vi "Usuarios-VI.vi"() -> (1 "Retroceder LED":bool, 2 "Estacionarse LED":bool)   [LabVIEW 2024]
uses:
  <vilib>/DAQmx/read.llb/DAQmx Read (Counter U32 1Chan 1Samp).vi
  <vilib>/DAQmx/miscellaneous.llb/DAQmx Fill In Error Info.vi
panel:
  in  "Retroceder":bool
  in  "Estacionarse":bool
  in  "Usuario invalido":T1={"Nombre de usuario"="Usuario NO Valido", "Nombre"="", "Fotografía"=FALSE}
  in  "Usuario 3":T1={"Nombre de usuario"="Yucateco_Belicon_27", "Nombre"="David Alejandro Zarazua Martinez", "Fotografía"=FALSE}
  in  "Usuario 1":T1={"Nombre de usuario"="Test_1", "Nombre"="Roberto Gomez Cruz", "Fotografía"=FALSE}
  in  "Usuario 2":T1={"Nombre de usuario"="El_Inge", "Nombre"="Ivan Nieto Guerrero", "Fotografía"=FALSE}
  out "Mensaje de entrada":string
  out "Credencial":u32
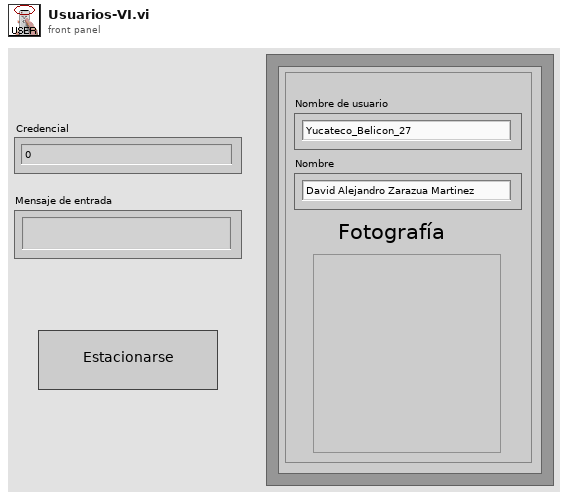
[diagram p1: front panel]
types:
  T1 = cluster{"Nombre de usuario":string, "Nombre":string, "Fotografía":bool}
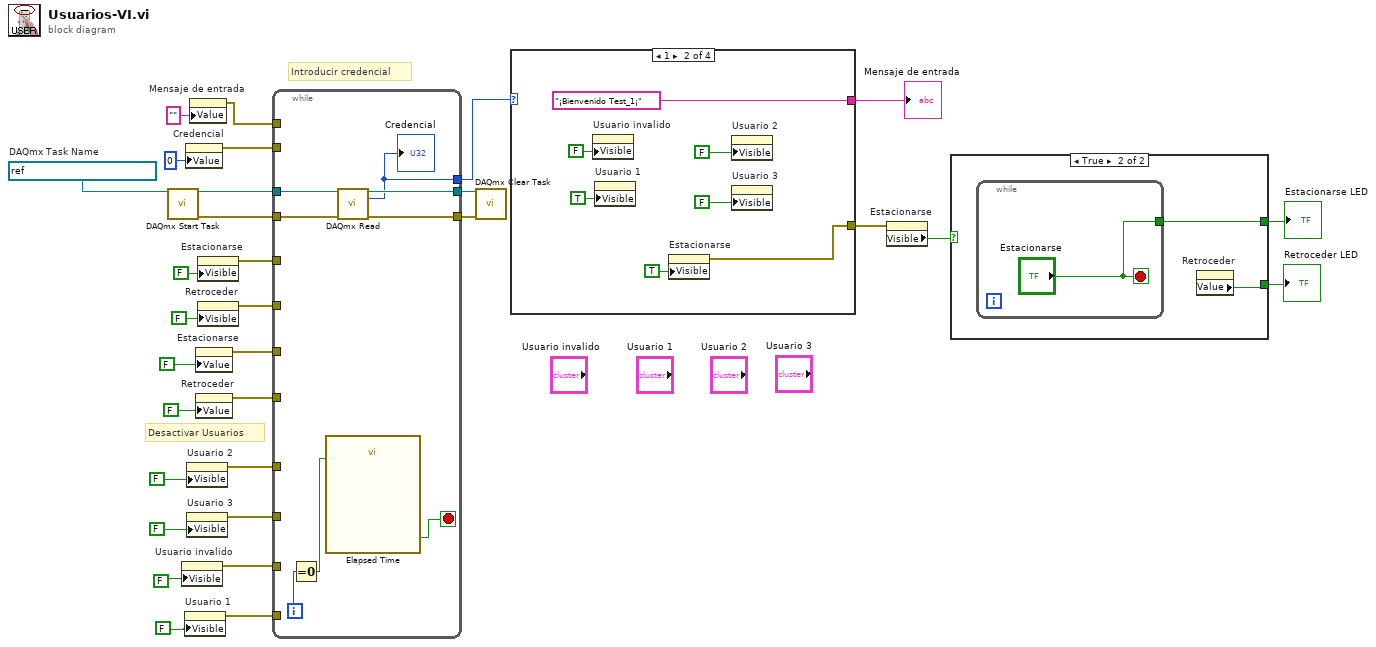
[diagram p0: block diagram]
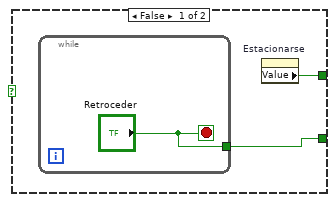
[diagram p2: hidden frame]
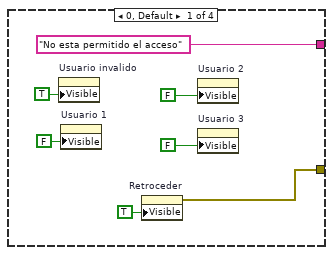
[diagram p3: hidden frame]
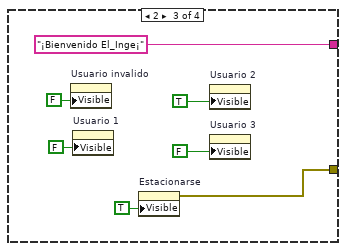
[diagram p4: hidden frame]
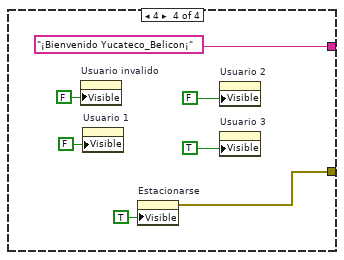
[diagram p5: hidden frame]
diagram:
  w31 = refnum<k21> "Contador de Pulso PF1"  # DAQmx Task Name
  # "Introducir credencial"
  # "Desactivar Usuarios"
  n1 = call <vilib>:"DAQmx Start Task.vi"("task/channels in"=w31) -> ("task out"=w30:refnum<k21>, "error out"=w29:errorcluster)  [unwired: 13 in]
  n2 = property on="Usuario invalido" class="Clust (strict)"("Visible"=FALSE) -> (error out=w18:errorcluster)  [unwired: 2 in, 1 out]
  n3 = property on="Usuario 1" class="Clust (strict)"("Visible"=FALSE) -> (error out=w17:errorcluster)  [unwired: 2 in, 1 out]
  n4 = property on="Credencial" class="DigNum (strict)"("Value"=u32 0 ("Credencial")) -> (error out=w14:errorcluster)  [unwired: 2 in, 1 out]
  n5 = property on="Usuario 2" class="Clust (strict)"("Visible"=FALSE) -> (error out=w23:errorcluster)  [unwired: 2 in, 1 out]
  n6 = property on="Usuario 3" class="Clust (strict)"("Visible"=FALSE) -> (error out=w24:errorcluster)  [unwired: 2 in, 1 out]
  n7 = property on="Mensaje de entrada" class="Str"("Value"="" ("Mensaje de entrada")) -> (error out=w13:errorcluster)  [unwired: 2 in, 1 out]
  n8 = property on="Estacionarse" class="Bool (strict)"("Value"=FALSE ("Estacionarse")) -> (error out=w6:errorcluster)  [unwired: 2 in, 1 out]
  n9 = property on="Retroceder" class="Bool (strict)"("Value"=FALSE ("Retroceder")) -> (error out=w5:errorcluster)  [unwired: 2 in, 1 out]
  n10 = property on="Estacionarse" class="Bool (strict)"("Visible"=FALSE) -> (error out=w8:errorcluster)  [unwired: 2 in, 1 out]
  n11 = property on="Retroceder" class="Bool (strict)"("Visible"=FALSE) -> (error out=w7:errorcluster)  [unwired: 2 in, 1 out]
  n12 = while {
    tunnel: w30 -> [w36]
    tunnel: w29 -> [w39]
    tunnel: [w37] -> w21
    tunnel: [w38] -> w20
    tunnel: [w35] -> w19
    tunnel: w24 -> [_]
    tunnel: w23 -> [_]
    tunnel: w18 -> [_]
    tunnel: w17 -> [_]
    tunnel: w14 -> [_]
    tunnel: w13 -> [_]
    tunnel: w8 -> [_]
    tunnel: w7 -> [_]
    tunnel: w6 -> [_]
    tunnel: w5 -> [_]
    i -> [w33]
    stop <- w34 stop-if-true
    n13 = Equal To 0?(x=w33) -> (x = 0?=w32:bool)
    n14 = call "Elapsed Time"("Reset"=w32) -> ("Time has Elapsed"=w34:bool)  [unwired: 11 in, 7 out]
    n15 = call-poly <vilib>:"DAQmx Read.vi"("task/channels in"=w36, "error in"=w39) -> ("task out"=w37:refnum<k21>, "data"=w35:u32, "error out"=w38:errorcluster)  [unwired: 11 in]
    "Credencial" <- w35
  }
  n16 = call <vilib>:"DAQmx Clear Task.vi"("task in"=w21, "error in"=w20) -> ()  [unwired: 13 in, 1 out]
  n17 = case shown="1" w19 {
    tunnel: ["No esta permitido el acceso" "¡Bienvenido Test_1¡" "¡Bienvenido El_Inge¡" "¡Bienvenido Yucateco_Belicon¡"] -> w10
    tunnel: [w40 w47 w54 w61] -> w9
    frame 0, Default {
      n18 = property on="Usuario invalido" class="Clust (strict)"("Visible"=TRUE) -> ()  [unwired: 2 in, 2 out]
      n19 = property on="Usuario 1" class="Clust (strict)"("Visible"=FALSE) -> ()  [unwired: 2 in, 2 out]
      n20 = property on="Retroceder" class="Bool (strict)"("Visible"=TRUE) -> (error out=w40:errorcluster)  [unwired: 2 in, 1 out]
      n21 = property on="Usuario 2" class="Clust (strict)"("Visible"=FALSE) -> ()  [unwired: 2 in, 2 out]
      n22 = property on="Usuario 3" class="Clust (strict)"("Visible"=FALSE) -> ()  [unwired: 2 in, 2 out]
    }
    frame 1 {
      n23 = property on="Usuario invalido" class="Clust (strict)"("Visible"=FALSE) -> ()  [unwired: 2 in, 2 out]
      n24 = property on="Usuario 1" class="Clust (strict)"("Visible"=TRUE) -> ()  [unwired: 2 in, 2 out]
      n25 = property on="Estacionarse" class="Bool (strict)"("Visible"=TRUE) -> (error out=w47:errorcluster)  [unwired: 2 in, 1 out]
      n26 = property on="Usuario 2" class="Clust (strict)"("Visible"=FALSE) -> ()  [unwired: 2 in, 2 out]
      n27 = property on="Usuario 3" class="Clust (strict)"("Visible"=FALSE) -> ()  [unwired: 2 in, 2 out]
    }
    frame 2 {
      n28 = property on="Usuario invalido" class="Clust (strict)"("Visible"=FALSE) -> ()  [unwired: 2 in, 2 out]
      n29 = property on="Usuario 1" class="Clust (strict)"("Visible"=FALSE) -> ()  [unwired: 2 in, 2 out]
      n30 = property on="Estacionarse" class="Bool (strict)"("Visible"=TRUE) -> (error out=w54:errorcluster)  [unwired: 2 in, 1 out]
      n31 = property on="Usuario 2" class="Clust (strict)"("Visible"=TRUE) -> ()  [unwired: 2 in, 2 out]
      n32 = property on="Usuario 3" class="Clust (strict)"("Visible"=FALSE) -> ()  [unwired: 2 in, 2 out]
    }
    frame 4 {
      n33 = property on="Usuario invalido" class="Clust (strict)"("Visible"=FALSE) -> ()  [unwired: 2 in, 2 out]
      n34 = property on="Usuario 1" class="Clust (strict)"("Visible"=FALSE) -> ()  [unwired: 2 in, 2 out]
      n35 = property on="Estacionarse" class="Bool (strict)"("Visible"=TRUE) -> (error out=w61:errorcluster)  [unwired: 2 in, 1 out]
      n36 = property on="Usuario 2" class="Clust (strict)"("Visible"=FALSE) -> ()  [unwired: 2 in, 2 out]
      n37 = property on="Usuario 3" class="Clust (strict)"("Visible"=TRUE) -> ()  [unwired: 2 in, 2 out]
    }
  }
  "Mensaje de entrada" <- w10
  n38 = property on="Estacionarse" class="Bool (strict)"(error in=w9) -> ("Visible"=w11:bool)  [unwired: 1 in, 2 out]
  n39 = case shown="True" w11 {
    tunnel: [w68 w72] -> w2
    tunnel: [w69 w71] -> w1
    frame False {
      n40 = while {
        tunnel: ["Retroceder"] -> w68
        stop <- "Retroceder" stop-if-true
      }
      n41 = property on="Estacionarse" class="Bool (strict)"() -> ("Value"=w69:bool)  [unwired: 2 in, 2 out]
    }
    frame True {
      n42 = while {
        tunnel: ["Estacionarse"] -> w71
        stop <- "Estacionarse" stop-if-true
      }
      n43 = property on="Retroceder" class="Bool (strict)"() -> ("Value"=w72:bool)  [unwired: 2 in, 2 out]
    }
  }
  "Estacionarse LED" <- w1
  "Retroceder LED" <- w2
